vi "Init_Hittite.vi"(0 "Serial configuration":T1={"Baud Rate"=9600, "Parity"=0, "Data Bits"=8, "Stop Bits"=10, "Flow Control"=0}, 2 "Com_port":refnum<visa-resource-name>, 3 "Trigger_channel":tag) -> (6 "Hittite_com":refnum<visa-resource-name>, 7 "Trigger_out":refnum<k21>, 8 "error out":errorcluster)   [LabVIEW 2014]
uses:
  <vilib>/DAQmx/write.llb/DAQmx Write (Digital Bool 1Line 1Point).vi
  <vilib>/DAQmx/create/channels.llb/DAQmx Create Channel (DO-Digital Output).vi
  <vilib>/DAQmx/miscellaneous.llb/DAQmx Fill In Error Info.vi
  D:/Microscope/Software/external_libraries/HMC-T2100/Private/Set source to Sweep Frequency .vi
  D:/Microscope/Software/external_libraries/HMC-T2100/Private/Set Sweep Direction Up.vi
  D:/Microscope/Software/external_libraries/HMC-T2100/Private/Go to Local.vi
  D:/Microscope/Software/external_libraries/HMC-T2100/HMC-T2100.lvlib
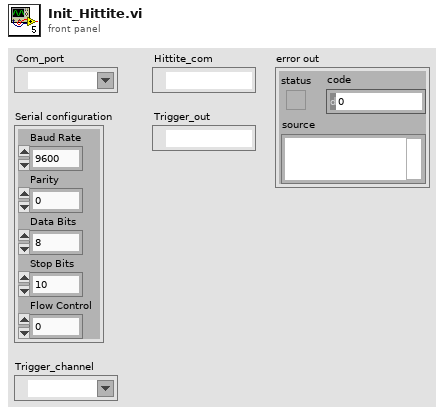
[diagram p1: front panel]
types:
  T1 = cluster{"Baud Rate":u32, "Parity":u16, "Data Bits":u16, "Stop Bits":u16, "Flow Control":u16}
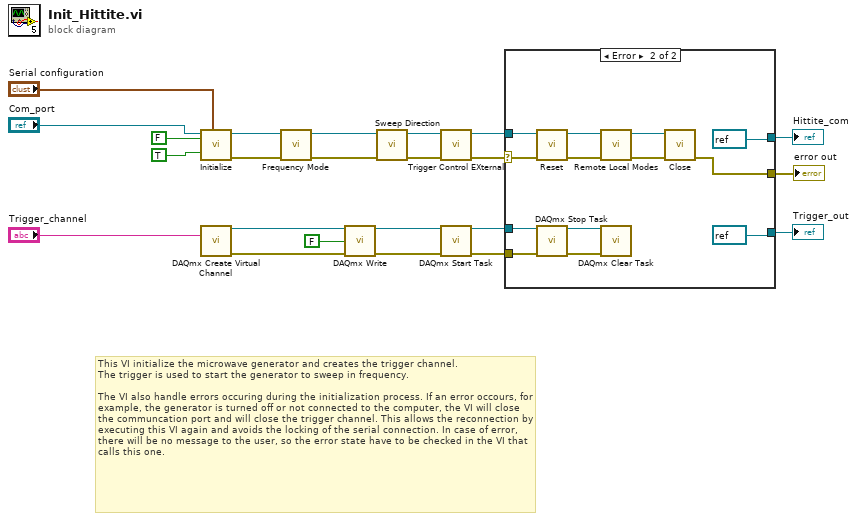
[diagram p0: block diagram]
diagram:
  # "This VI initialize the microwave generator and creates the trigger channel.\nThe trigger is used to start the generator to sweep in frequency.\n\nThe VI also handle errors occuring during the initialization process. If an error occours, for example, the generator is turned off or not connected to the computer, the VI will close the communcation port and will close the trigger channel. This allows the reconnection by executing this VI again and avoids the locking of the serial connection. In case of error, there will be no message to the user, so the error state have to be checked in the VI that calls this one."
  n1 = call "Initialize.vi"("Serial Configuration"="Serial configuration", "Reset (True)"=TRUE, "ID Query (True)"=FALSE, "VISA resource name"="Com_port") -> ("error out"=w12:errorcluster, "VISA resource name out"=w21:refnum<visa-resource-name>)  [unwired: 6 in]
  n2 = call-poly <vilib>:"DAQmx Create Virtual Channel.vi"("lines"="Trigger_channel") -> ("task out"=w18:refnum<k21>, "error out"=w3:errorcluster)  [unwired: 13 in]
  n3 = call-poly "Frequency Mode.vi"("error in"=w12, "T2100 Address IN"=w21) -> ("error out"=w11:errorcluster, "T2100 Address OUT"=w22:refnum<visa-resource-name>)  [unwired: 8 in]
  n4 = call-poly <vilib>:"DAQmx Write.vi"("task/channels in"=w18, "data"=FALSE, "error in"=w3) -> ("task out"=w20:refnum<k21>, "error out"=w2:errorcluster)  [unwired: 10 in, 1 out]
  n5 = call-poly "Sweep Direction.vi"("error in"=w11, "VISA resource name"=w22) -> ("error out"=w10:errorcluster, "VISA resource name out"=w23:refnum<visa-resource-name>)  [unwired: 8 in]
  n6 = call "Trigger Control EXternal.vi"("error in"=w10, "T2100 Address In"=w23) -> ("error out"=w9:errorcluster, "T2100 Address Out"=w8:refnum<visa-resource-name>)  [unwired: 8 in]
  n7 = call <vilib>:"DAQmx Start Task.vi"("task/channels in"=w20, "error in"=w2) -> ("task out"=w7:refnum<k21>, "error out"=w1:errorcluster)  [unwired: 12 in]
  n8 = case shown="Error" w9 {
    selector: w9 -> [w24 w32]
    tunnel: w8 -> [w26 w33]
    tunnel: w7 -> [w25 w38]
    tunnel: [w26 refnum<visa-resource-name> refnum ("T2100 Address Out")] -> w6
    tunnel: [w25 refnum<k21> refnum ("task out")] -> w5
    tunnel: [w24 w31] -> w4
    tunnel: w1 -> [_ w28]
    frame No Error {
    }
    frame Error {
      n9 = call "Reset.vi"("error in"=w32, "T2100 Address In"=w33) -> ("error out"=w36:errorcluster, "T2100 Address Out"=w35:refnum<visa-resource-name>)  [unwired: 8 out]
      n10 = call <vilib>:"DAQmx Stop Task.vi"("task/channels in"=w38, "error in"=w28) -> ("task out"=w39:refnum<k21>, "error out"=w27:errorcluster)  [unwired: 12 in]
      n11 = call-poly "Remote Local Modes.vi"("error in"=w36, "T2100 Address In"=w35) -> ("error out"=w37:errorcluster, "T2100 Address Out"=w34:refnum<visa-resource-name>)  [unwired: 8 in]
      n12 = call <vilib>:"DAQmx Clear Task.vi"("task in"=w39, "error in"=w27) -> ()  [unwired: 13 in, 1 out]
      n13 = call "Close.vi"("error in (no error)"=w37, "VISA resource name"=w34) -> ("error out"=w31:errorcluster)  [unwired: 9 in]
    }
  }
  "Trigger_out" <- w5
  "Hittite_com" <- w6
  "error out" <- w4
